vi "FTPData.vi"(4 "POP params":T1, 5 "FTP params":T2, 7 "directory path":path=path "D:/") -> ()   [LabVIEW 2022 SP3]
uses:
  <vilib>/Utility/SMTP/NI_SMTPEmail.lvlib
  <vilib>/FTP/NI_FTP.lvlib
panel:
  out "TIme":u8(slide) scale=0.0..100.0
  out "spreadsheet string":string
  # "FTP in progress. Report errors to RRI."
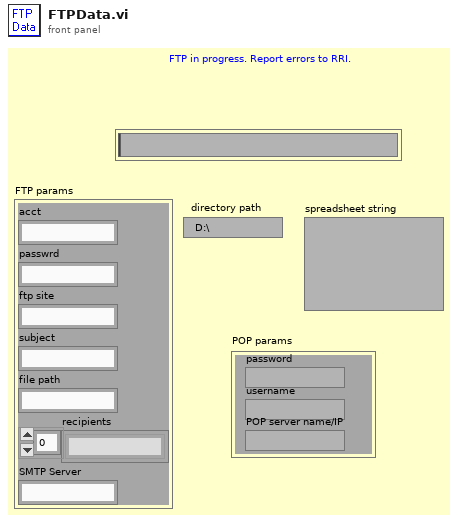
[diagram p1: front panel]
types:
  T1 = cluster{"password":string, "username":string, "POP server name/IP":string}
  T2 = cluster{"acct":string, "passwrd":string, "ftp site":string, "subject":string, "file path":string, "recipients":string[], "SMTP Server":string}
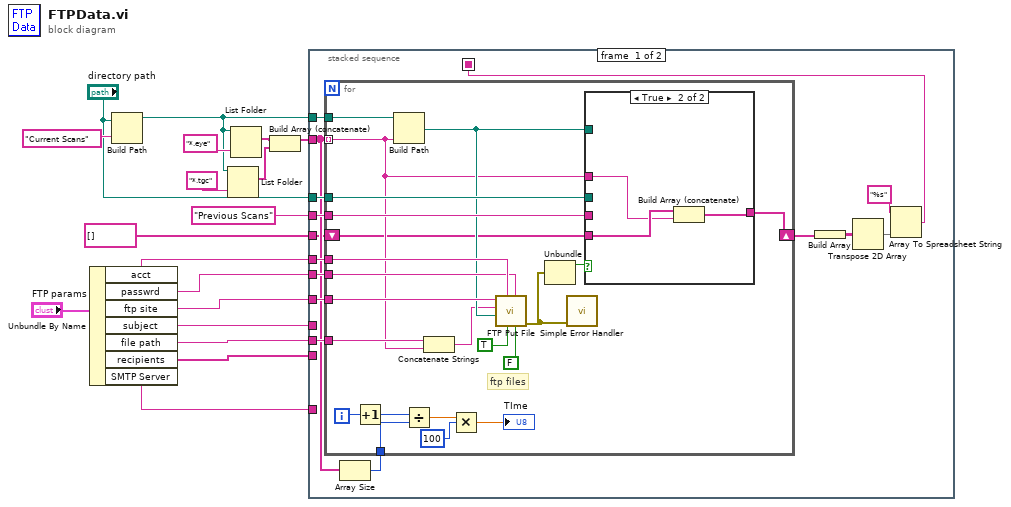
[diagram p0: block diagram]
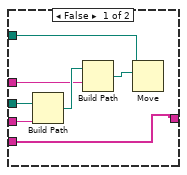
[diagram p2: hidden frame]
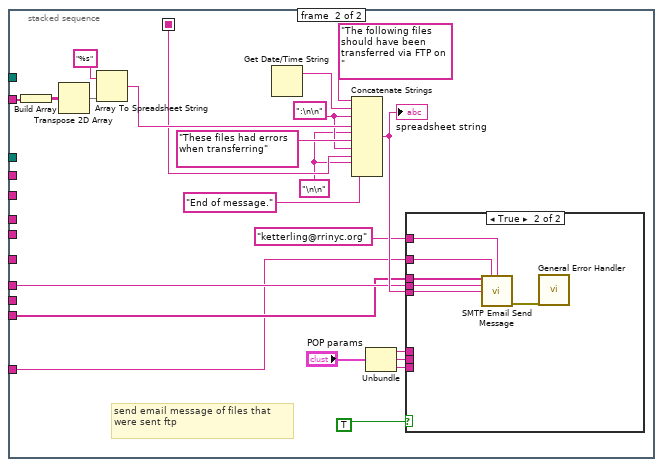
[diagram p3: hidden frame]
diagram:
  n1 = Unbundle By Name("FTP params") -> ("acct"=w8:string, "passwrd"=w7:string, "ftp site"=w6:string, "subject"=w5:string, "file path"=w4:string, "recipients"=w3:string[], "SMTP Server"=w2:string)
  n2 = Build Path(base path="directory path", name or relative path="Current Scans") -> (appended path=w12:path)
  n3 = List Folder(path=w12, pattern="*.tgc") -> (filenames=w14:string[])  [unwired: 2 in, 3 out]
  n4 = List Folder(path=w12, pattern="*.eye") -> (filenames=w15:string[])  [unwired: 2 in, 3 out]
  n5 = Build Array (concatenate)(w15, w14) -> (w13:string[])
  n6 = stacked-sequence {
    seq-local: [w19 _] -> [_ w72]
    tunnel: "Previous Scans" -> [w33 _]
    tunnel: w12 -> [w32 _]
    tunnel: w13 -> [w26 w87]
    tunnel: w4 -> [w31 _]
    tunnel: w8 -> [w30 _]
    tunnel: w7 -> [w29 _]
    tunnel: w5 -> [_ w79]
    tunnel: w6 -> [w27 _]
    tunnel: "directory path" -> [w28 _]
    tunnel: w3 -> [_ w78]
    tunnel: w2 -> [_ w77]
    tunnel: string[] [] -> [w24 _]
    frame #0 {
      n7 = Array Size(array=w26) -> (size(s)=w25:i32)
      n8 = for {
        tunnel: w26 -> [w47] mode=indexing
        tunnel: w32 -> [w52]
        tunnel: w33 -> [w50]
        tunnel: w31 -> [w55]
        tunnel: w30 -> [w54]
        tunnel: w29 -> [w53]
        tunnel: w28 -> [w49]
        tunnel: w27 -> [w51]
        tunnel: w25 -> [w37]
        shift-right: [w36] -> w21
        shift-left: w24 -> [w35]
        i -> [w42]
        # "ftp files"
        n9 = Increment(x=w42) -> (x+1=w38:i32)
        n10 = Build Path(base path=w52, name or relative path=w47) -> (appended path=w48:path)
        n11 = Divide(x=w38, y=w37) -> (x/y=w41:dbl)
        n12 = Concatenate Strings(w55, w47) -> (w45:string)
        n13 = Multiply(x=w41, y=100) -> (x*y=→"TIme":dbl)
        n14 = call <vilib>:"FTP Put File.vi"("active (T)"=FALSE ("binary (F)"), "password"=w53, "binary (F)"=TRUE, "user"=w54, "local path"=w48, "remote path"=w45, "host"=w51) -> ("error out"=w34:errorcluster)  [unwired: 3 in, 1 out]
        n15 = Unbundle(w34) -> ("status"=w44:bool)  [unwired: 2 out]
        n16 = call <vilib>:"Simple Error Handler.vi"("error in (no error)"=w34) -> ()  [unwired: 4 in, 5 out]
        n17 = case shown="True" w44 {
          tunnel: w50 -> [w60 _]
          tunnel: w49 -> [w59 _]
          tunnel: w48 -> [w58 _]
          tunnel: w47 -> [w57 w64]
          tunnel: [w56 w63] -> w36
          tunnel: w35 -> [w56 w65]
          frame False {
            n18 = Build Path(base path=w59, name or relative path=w60) -> (appended path=w62:path)
            n19 = Build Path(base path=w62, name or relative path=w57) -> (appended path=w61:path)
            n20 = Move(source path=w58, 10:w61) -> ()  [unwired: 3 in, 3 out]
          }
          frame True {
            n21 = Build Array (concatenate)(w65, w64) -> (w63:string[])
          }
        }
      }
      n22 = Build Array(w21) -> (w23:string[][])
      n23 = Transpose 2D Array(2D array=w23) -> (transposed array=w22:string[][])
      n24 = Array To Spreadsheet String(array=w22, 3:"%s" ("format string")) -> (spreadsheet string=w19:string)  [unwired: 1 in]
    }
    frame #1 {
      w71 = "\n\n"
      w73 = ":\n\n"
      # "send email message of files that were sent ftp"
      n25 = Build Array(w87) -> (w86:string[][])
      n26 = Transpose 2D Array(2D array=w86) -> (transposed array=w84:string[][])
      n27 = Array To Spreadsheet String(array=w84, 3:"%s" ("format string")) -> (spreadsheet string=w82:string)  [unwired: 1 in]
      n28 = Get Date/Time String() -> (date string=w75:string)  [unwired: 3 in, 1 out]
      n29 = Concatenate Strings("The following files should have been transferred via FTP on ", w75, w73, w82, w71, "These files had errors when transferring", w73, w72, w71, "End of message.") -> (w81:string)
      "spreadsheet string" <- w81
      n30 = Unbundle("POP params") -> ("password"=w68:string, "username"=w67:string, "POP server name/IP"=w66:string)
      n31 = case shown="True" TRUE ("Case Constant\n(See Context Help)") {
        tunnel: w81 -> [_ w93]
        tunnel: "ketterling@rrinyc.org" -> [_ w92]
        tunnel: w79 -> [_ w91]
        tunnel: w78 -> [_ w90]
        tunnel: w77 -> [_ w89]
        tunnel: w68 -> [_ _]
        tunnel: w67 -> [_ _]
        tunnel: w66 -> [_ _]
        frame False {
        }
        frame True {
          n32 = call <vilib>:"SMTP Email Send Message.vi"("recipients"=w90, "mail server"=w89, "return address"=w92, "subject ([No Subject])"=w91, "message"=w93) -> ("error out"=w88:errorcluster)  [unwired: 9 in, 1 out]
          n33 = call <vilib>:"General Error Handler.vi"("error in (no error)"=w88) -> ()  [unwired: 10 in, 5 out]
        }
      }
    }
  }
